vi "APC_PC_PythonGateway.vi"() -> ()   [LabVIEW 2020]
uses:
  controls/APC_ControlSettings.ctl
  controls/APC_PIDcontrolSettings.ctl
panel:
  out "System State 2":i8
  in  "stop":bool
  out "Client Connected":bool=TRUE
  out "Telemetry seq":i32
  out "Lines received":i32
  out "Last received":string
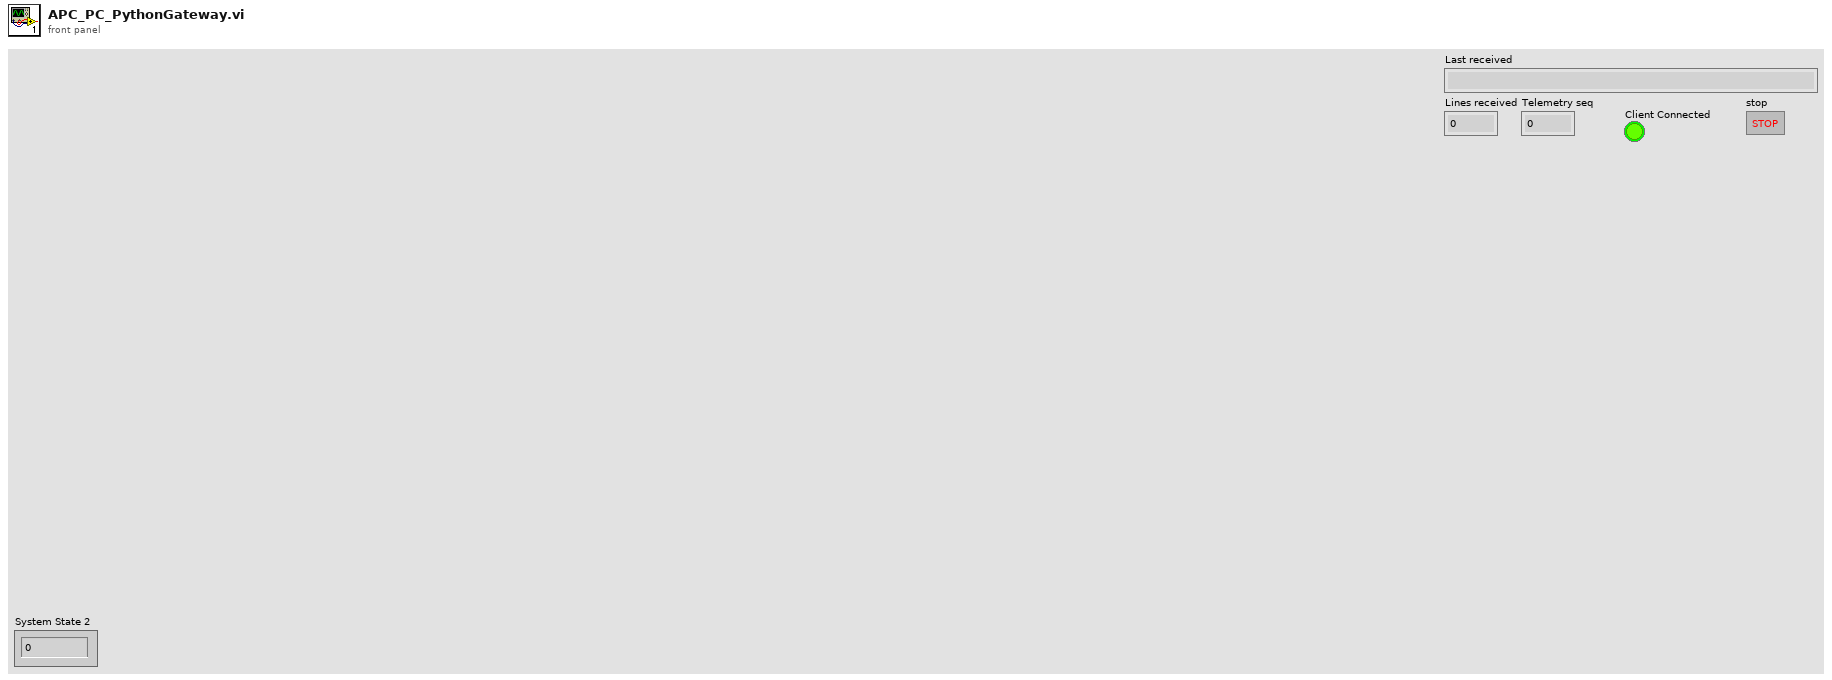
[diagram p1: front panel]
types:
  T1 = enum16{"Standard", "Buffered", "CRLF", "Immediate"}
  T2 = typedef "APC_ControlSettings.ctl" = cluster{"Spark advance [CADBTDC]":dbl, "Pref":dbl, "O2ref":dbl, "DI advance [CADBTDC]":dbl, "DI duration [ms] ":dbl, "CO2ref":dbl, "PFI duration [ms]":dbl, "IMEP ref":dbl, "Speed ref":dbl, "IGN enable":bool, "DI enable":bool, "CL PFI\n lambda":bool, "CL PFI\nIMEP":bool, "Activate\ncylinder":bool[], "Force idling":bool, "Force motoring":bool, "ETP resync":bool, "Requested mode":i8, "Clear Sync Errors":bool, "toggle TDC":bool, "l ref":dbl, "PID control references":T3, "CA50setpoint [CADATDC]":dbl, "CA50 control":bool, "Knock control":bool, "CLEAR EMERGENCY STOP":bool, "EMERGENCY STOP":bool}
  T3 = typedef "APC_PIDcontrolSettings.ctl" = cluster{"NG":bool, "Ar":bool, "O2":bool, "Intake vent":bool, "Cross vent":bool, "Exhaust vent":bool, "NG control mode":u8, "NG-FC-001-REF":dbl, "WF-OA-002-REF":dbl, "IMEP-REF":dbl, "Nm-REF":dbl, "Ar control mode":u8, "AR-PC-002-REF":dbl, "WF-PT-004-REF":dbl, "O2 control mode":u8, "O2-FC-001-REF":dbl, "WF-OA-001-REF":dbl, "Tcoolant control  mode":u8, "EC-FC-001-REF":dbl, "EC-TT-001-REF":dbl, "Texh control mode":u8, "SW-FC-004-REF":dbl, "SW-FT-002-REF":dbl, "WF-TT-004-REF":dbl, "Toil control mode":u8, "SW-FC-009-REF":dbl, "SW-FT-004-REF":dbl, "EO-TT-001-REF":dbl, "AIC201_CO2_ConcTarget":dbl, "O2_FF_NG":bool, "Dyno control mode":u8, "Membrane control mode":u8, "AR-FT-001-REF":dbl, "MTR modbus floats":sgl[], "MTR modbus u16":u16[], "MTR HB":bool, "PC_HB":bool, "EMERGENCY STOP":bool}
  T4 = cluster{"Spark advance [CADBTDC]":dbl, "Pref":dbl, "O2ref":dbl, "DI advance [CADBTDC]":dbl, "DI duration [ms] ":dbl, "CO2ref":dbl, "PFI duration [ms]":dbl, "IMEP ref":dbl, "Speed ref":dbl, "IGN enable":bool, "DI enable":bool, "CL PFI\n lambda":bool, "CL PFI\nIMEP":bool, "Activate\ncylinder":bool[], "Force idling":bool, "Force motoring":bool, "ETP resync":bool, "Requested mode":i8, "Clear Sync Errors":bool, "toggle TDC":bool, "l ref":dbl, "PID control references":T3, "CA50setpoint [CADATDC]":dbl, "CA50 control":bool, "Knock control":bool, "CLEAR EMERGENCY STOP":bool, "EMERGENCY STOP":bool}
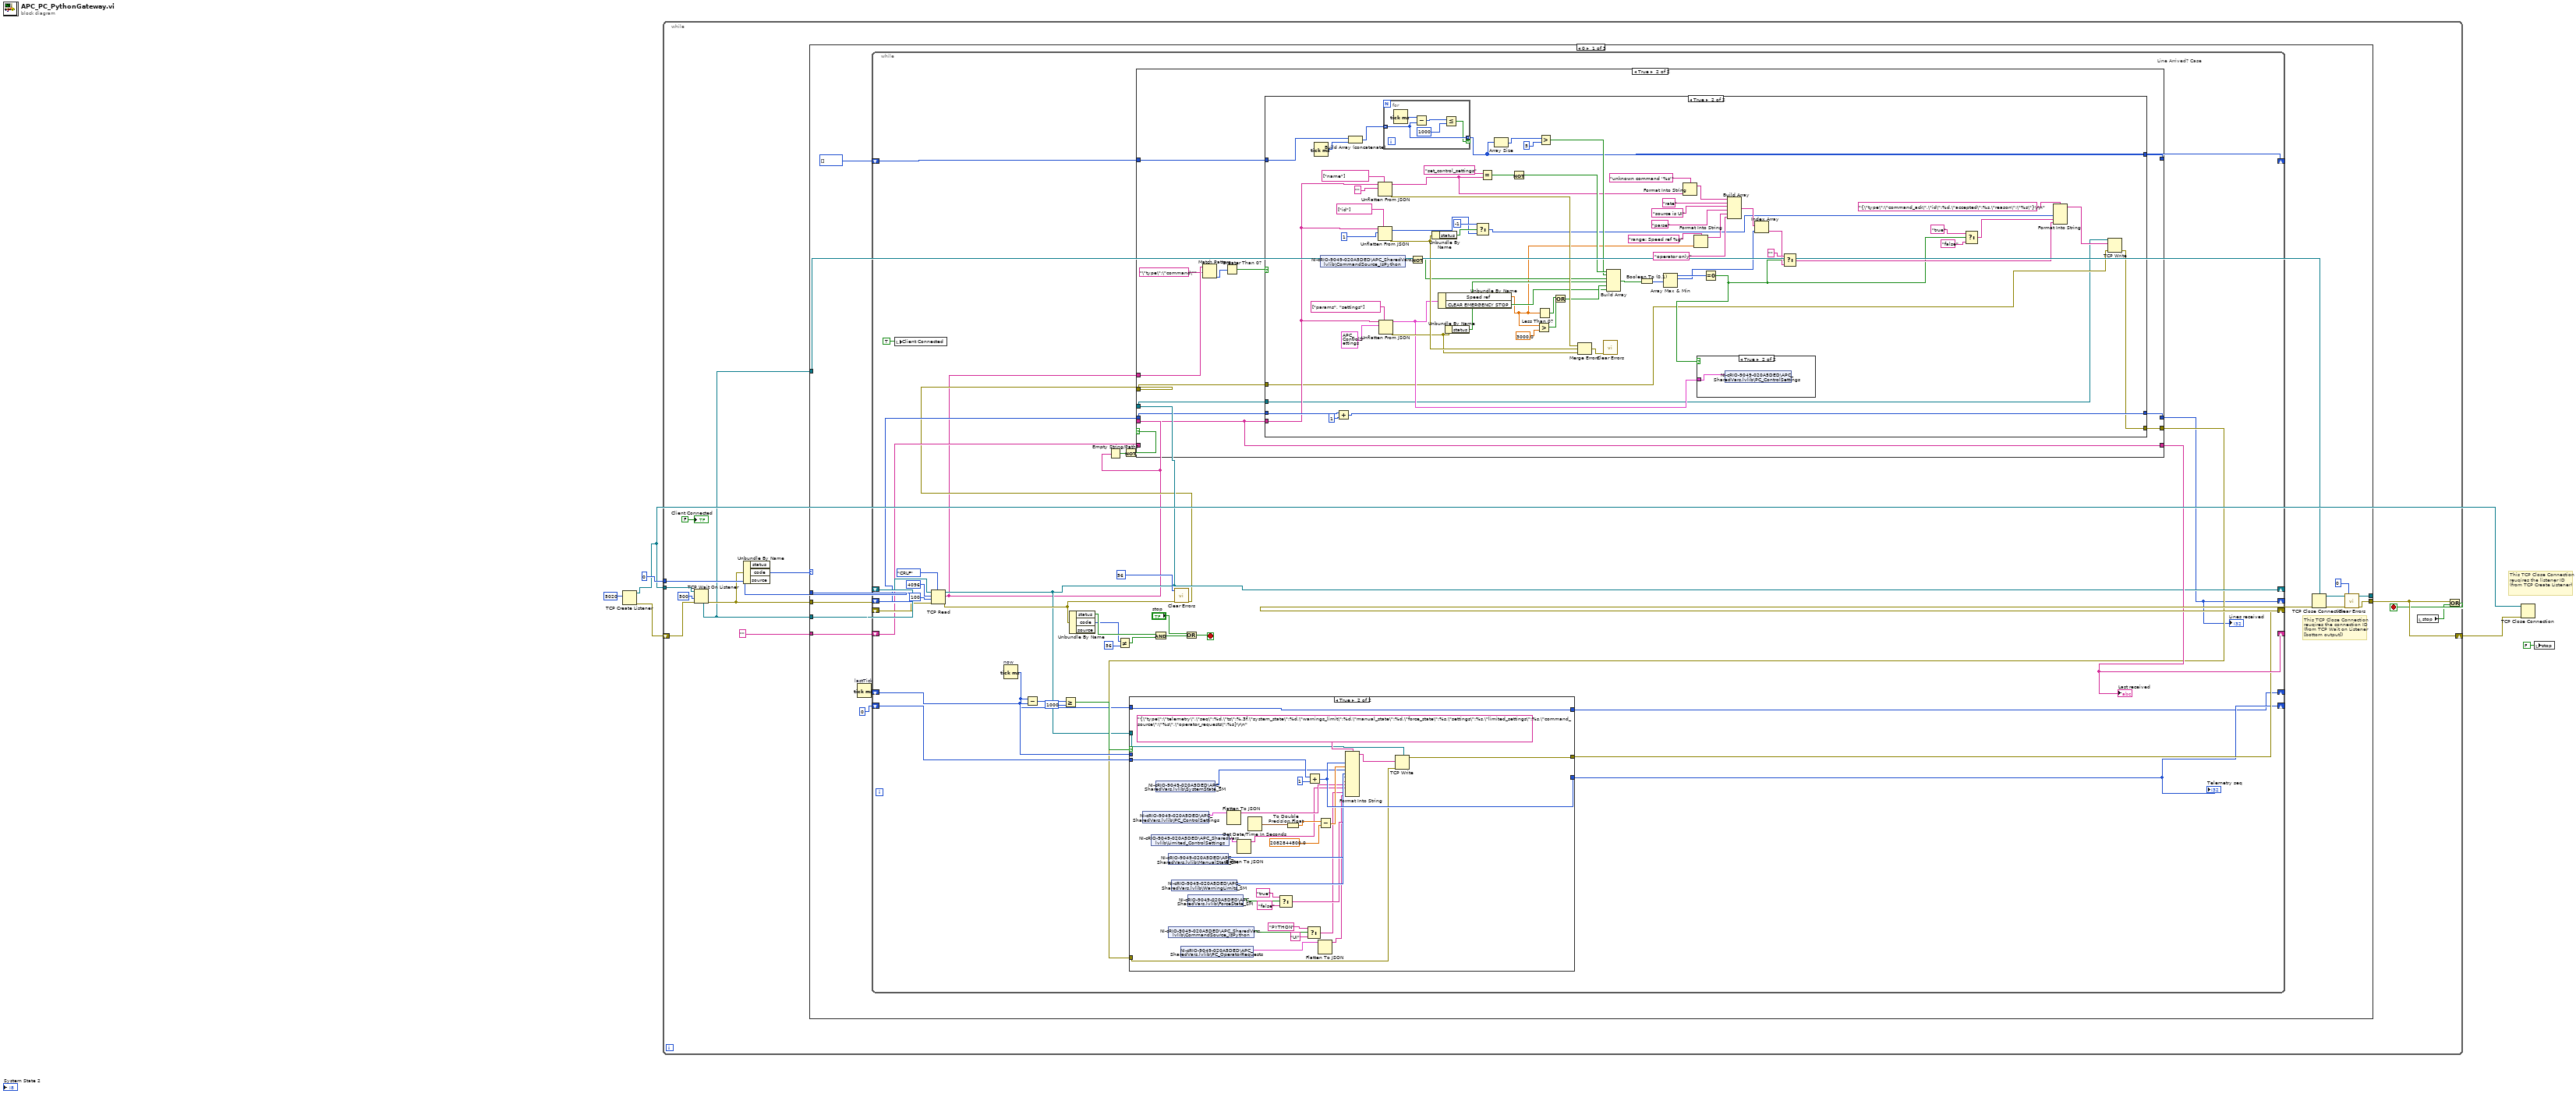
[diagram p0: block diagram]
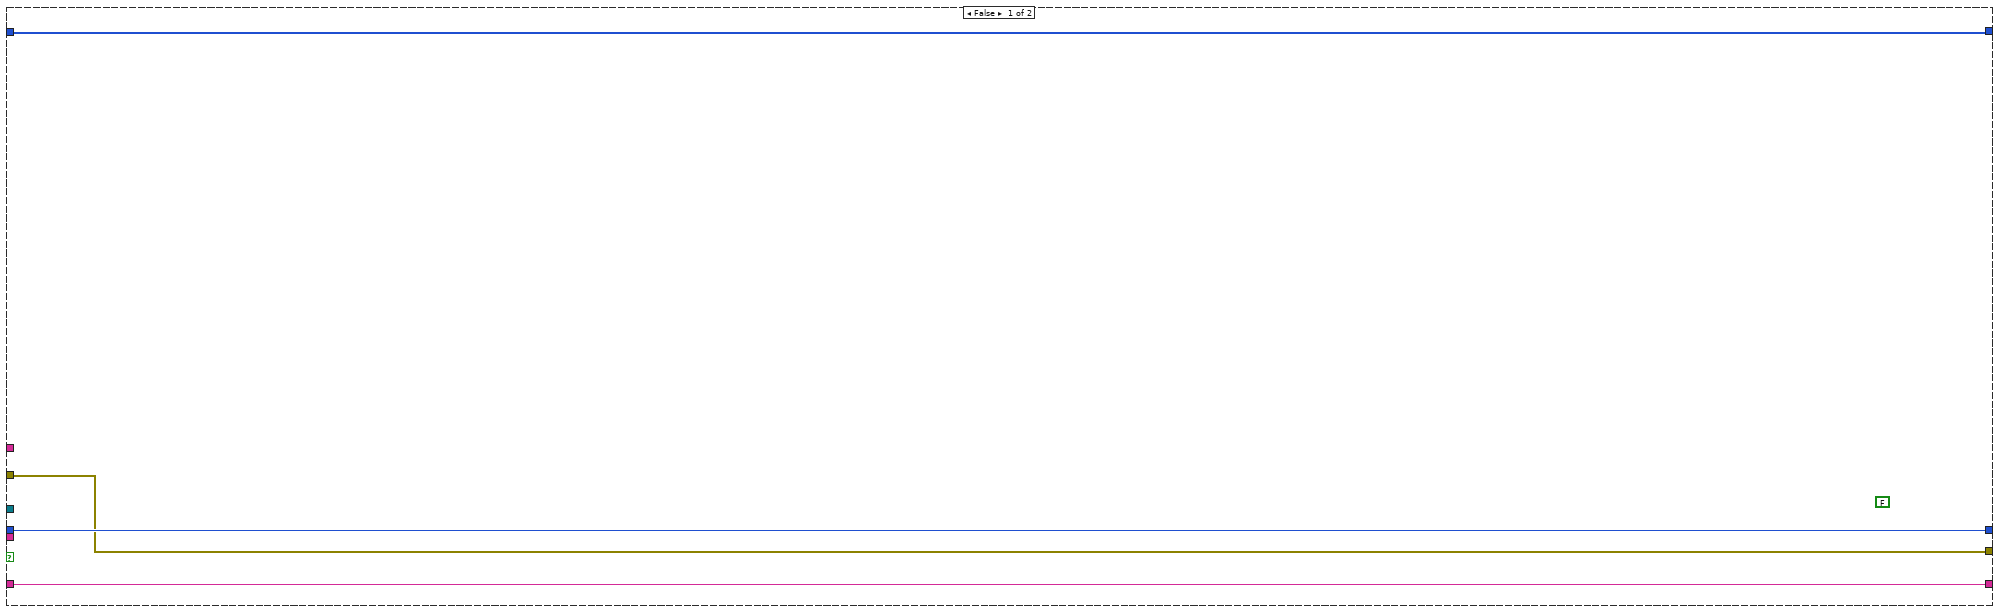
[diagram p3: hidden frame]
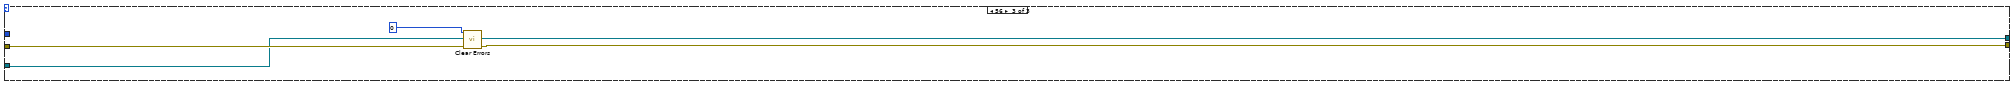
[diagram p7: hidden frame]
diagram:
  # "This TCP Close Connection reuqires the listener ID (from TCP Create Listener)"
  n1 = TCP Create Listener(10:u16 5020 ("port")) -> (0:w4:errorcluster, 3:w1:refnum<k5>)  [unwired: 4 in, 1 out]
  n2 = while {
    tunnel: 0 ("Lines received") -> [w17]
    shift-right: [w12] -> w3
    shift-left: w4 -> [w16]
    tunnel: w1 -> [w9]
    stop <- w11 stop-if-true
    n3 = TCP Wait On Listener(8:w16, 9:500 ("timeout ms (wait forever: -1)"), 11:w9) -> (0:w14:errorcluster, 4:w8:refnum<k5>)  [unwired: 1 in, 3 out]
    n4 = Unbundle By Name(w14) -> ("code"=w13:i32)  [unwired: 2 out]
    n5 = case shown="0" w13 {
      tunnel: w8 -> [w31 w191 w192]
      tunnel: w17 -> [w30 _ _]
      tunnel: [w24 w191 w192] -> _
      tunnel: [w25 w190 w193] -> w12
      tunnel: w14 -> [w29 w190 w194]
      tunnel: w8 -> [w23 _ _]
      tunnel: "" -> [w22 _ _]
      frame 0 {
        # "This TCP Close Connection reuqires the connection ID (from TCP Wait on Listener [bottom output])"
        n6 = Tick Count (ms) "lastTick"() -> (millisecond timer value=w21:u32)
        n7 = while {
          shift-right: [w33] -> _
          shift-left: w30 -> [w58]
          shift-right: [w53] -> w28
          shift-left: w29 -> [w61]
          shift-right: [w38] -> _
          shift-left: w31 -> [w67]
          shift-right: [w59] -> _
          shift-left: w22 -> [w60]
          shift-right: [w51] -> _
          shift-left: w21 -> [w50]
          shift-right: [w52] -> _
          shift-left: 0 -> [w54]
          shift-right: [w39] -> _
          shift-left: u32[] [] -> [w40]
          stop <- w47 stop-if-true
          n8 = local write "Client Connected"(TRUE ("Client Connected")) -> ()
          n9 = TCP Read(connection ID=w67, bytes to read=4096, error in (no error)=w61, 7:T1."CRLF" ("mode (standard)"), 9:100 ("timeout ms (25000)")) -> (connection ID out=w38:refnum<k5>, data out=w32:string, error out=w48:errorcluster)
          n10 = Tick Count (ms) "now"() -> (millisecond timer value=w49:u32)
          n11 = Subtract(x=w49, y=w50) -> (x-y=w57:u32)
          n12 = Greater Or Equal?(x=w57, y=u32 1000) -> (x >= y?=w55:bool)
          n13 = Unbundle By Name(w48) -> ("status"=w44:bool, "code"=w43:i32)  [unwired: 1 out]
          n14 = Empty String/Path?(string/path=w32) -> (empty?=w35:bool)
          n15 = Not Equal?(x=w43, y=56) -> (x != y?=w41:bool)
          n16 = Not(x=w35) -> (.not. x?=w34:bool)
          n17 = And(x=w44, y=w41) -> (x .and. y?=w45:bool)
          n18 = call <vilib>:"Clear Errors.vi"("error in (no error)"=w48, "specific error code to clear (0: all)"=56) -> ("error out"=w37:errorcluster)  [unwired: 4 in, 1 out]
          n19 = case "Line Arrived? Case" shown="True" w34 {
            tunnel: w60 -> [w104 _]
            tunnel: [w104 w112] -> w59
            tunnel: w32 -> [_ w112]
            tunnel: w58 -> [w103 w116]
            tunnel: [w103 w115] -> w33
            tunnel: [w102 w113] -> w39
            tunnel: w40 -> [w102 w114]
            tunnel: w38 -> [_ w109]
            tunnel: w37 -> [w101 w110]
            tunnel: [w101 w111] -> w36
            tunnel: w32 -> [_ w107]
            frame False {
              (unwired) FALSE
            }
            frame True {
              n20 = Match Pattern(string=w107, regular expression="\"type\":\"command\"") -> (offset past match=w108:i32)  [unwired: 1 in, 3 out]
              n21 = Greater Than 0?(x=w108) -> (x > 0?=w105:bool)
              n22 = case shown="True" w105 {
                tunnel: w116 -> [w118 w182]
                tunnel: [w118 w181] -> w115
                tunnel: w114 -> [w117 w157]
                tunnel: [w117 w154] -> w113
                tunnel: w112 -> [_ w134]
                tunnel: [w119 w125] -> w111
                tunnel: w110 -> [w119 w124]
                tunnel: w109 -> [_ w123]
                frame False {
                }
                frame True {
                  n23 = Tick Count (ms)() -> (millisecond timer value=w156:u32)
                  n24 = shared-variable "NI-cRIO-9049-020A5DED\\APC_SharedVars.lvlib\\CommandSource_IsPython"() -> (w153:bool)  [unwired: 1 in, 1 out]
                  n25 = Add(x=w182, y=1) -> (x+y=w181:i32)
                  n26 = Build Array (concatenate)(w157, w156) -> (w155:u32[])
                  n27 = Unflatten From JSON(path=string[] ["id"], JSON string=w134, type and defaults=1 ("y")) -> (value=w171:i32, error out=w169:errorcluster)  [unwired: 4 in]
                  n28 = Unflatten From JSON(path=string[] ["name"], JSON string=w134, type and defaults="") -> (value=w146:string, error out=w170:errorcluster)  [unwired: 4 in]
                  n29 = Unflatten From JSON(path=string[] ["params", "settings"], JSON string=w134, type and defaults=T2 {"Spark advance [CADBTDC]"=0.0, "Pref"=0.0, "O2ref"=0.0, "DI advance [CADBTDC]"=0.0, "DI duration [ms] "=0.0, "CO2ref"=0.0, "PFI duration [ms]"=0.0, "IMEP ref"=0.0, "Speed ref"=1800.0, "IGN enable"=TRUE, "DI enable"=TRUE, "CL PFI\n lambda"=FALSE, "CL PFI\nIMEP"=FALSE, "Activate\ncylinder"=[FALSE, FALSE, FALSE, FALSE, FALSE, FALSE], "Force idling"=FALSE, "Force motoring"=FALSE, "ETP resync"=FALSE, "Requested mode"=0, "Clear Sync Errors"=FALSE, "toggle TDC"=FALSE, "l ref"=0.0, "PID control references"={"NG"=FALSE, "Ar"=FALSE, "O2"=FALSE, "Intake vent"=FALSE, "Cross vent"=FALSE, "Exhaust vent"=FALSE, "NG control mode"=0, "NG-FC-001-REF"=0.0, "WF-OA-002-REF"=0.0, "IMEP-REF"=0.0, "Nm-REF"=0.0, "Ar control mode"=0, "AR-PC-002-REF"=0.0, "WF-PT-004-REF"=0.0, "O2 control mode"=0, "O2-FC-001-REF"=0.0, "WF-OA-001-REF"=0.0, "Tcoolant control  mode"=0, "EC-FC-001-REF"=0.0, "EC-TT-001-REF"=0.0, "Texh control mode"=0, "SW-FC-004-REF"=0.0, "SW-FT-002-REF"=0.0, "WF-TT-004-REF"=0.0, "Toil control mode"=0, "SW-FC-009-REF"=0.0, "SW-FT-004-REF"=0.0, "EO-TT-001-REF"=0.0, "AIC201_CO2_ConcTarget"=0.0, "O2_FF_NG"=FALSE, "Dyno control mode"=0, "Membrane control mode"=0, "AR-FT-001-REF"=0.0, "MTR modbus floats"=[0.0, 0.0, 0.0, 0.0, 0.0, 0.0, 0.0, 0.0, 0.0, 0.0, 0.0, 0.0, 0.0, 0.0, 0.0, 0.0, 0.0, 0.0, 0.0], "MTR modbus u16"=[0, 0, 0, 0, 0, 0, 0], "MTR HB"=FALSE, "PC_HB"=FALSE, "EMERGENCY STOP"=FALSE}, "CA50setpoint [CADATDC]"=0.0, "CA50 control"=TRUE, "Knock control"=FALSE, "CLEAR EMERGENCY STOP"=FALSE, "EMERGENCY STOP"=FALSE} ("APCControlSettings")) -> (value=w133:T2, error out=w168:errorcluster)  [unwired: 4 in]
                  n30 = for {
                    tunnel: w155 -> [w186] mode=indexing
                    tunnel: [w186] -> w154 mode=indexing if=w185
                    n31 = Tick Count (ms)() -> (millisecond timer value=w189:u32)
                    n32 = Subtract(x=w189, y=w186) -> (x-y=w188:u32)
                    n33 = Less Or Equal?(x=w188, y=u32 1000) -> (x <= y?=w185:bool)
                  }
                  n34 = Not(x=w153) -> (.not. x?=w152:bool)
                  n35 = Unbundle By Name(w169) -> ("status"=w173:bool)
                  n36 = Unbundle By Name(w133) -> ("Speed ref"=w145:dbl, "CLEAR EMERGENCY STOP"=w150:bool)
                  n37 = Unbundle By Name(w168) -> ("status"=w164:bool)
                  n38 = Select(t=-1, s=w173, f=w171) -> (s? t:f=w131:i32)
                  n39 = Equal?(x="set_control_settings", y=w146) -> (x = y?=w166:bool)
                  n40 = Array Size(array=w154) -> (size(s)=w162:i32)
                  n41 = Not(x=w166) -> (.not. x?=w165:bool)
                  n42 = Greater?(x=w145, y=3000.0) -> (0:w158:bool)
                  n43 = Less Than 0?(x=w145) -> (x < 0?=w160:bool)
                  n44 = Greater?(x=w162, y=5) -> (0:w161:bool)
                  n45 = Or(x=w160, y=w158) -> (x .or. y?=w159:bool)
                  n46 = Merge Errors(w170, w169, w168) -> (w167:errorcluster)
                  n47 = call <vilib>:"Clear Errors.vi"("error in (no error)"=w167) -> ()  [unwired: 5 in, 2 out]
                  n48 = Build Array(w165, w161, w152, w164, w159, w150) -> (w149:bool[])
                  n49 = Boolean To (0,1)(Boolean=w149) -> (0, 1=w148:i16[])
                  n50 = Array Max & Min(array=w148) -> (max value=w147:i16, max index (indices)=w137:i32)  [unwired: 2 out]
                  n51 = Format Into String(format string="unknown command '%s'" ("initial string"), w146) -> (resulting string=w144:string)  [unwired: 2 in, 1 out]
                  n52 = Format Into String(format string="range: Speed ref %g" ("initial string"), w145) -> (resulting string=w140:string)  [unwired: 2 in, 1 out]
                  n53 = Equal To 0?(x=w147) -> (x = 0?=w130:bool)
                  n54 = case shown="True" w130 {
                    tunnel: w133 -> [_ w184]
                    frame False {
                    }
                    frame True {
                      n55 = shared-variable "NI-cRIO-9049-020A5DED\\APC_SharedVars.lvlib\\PC_ControlSettings"(w184) -> ()  [unwired: 1 in, 1 out]
                    }
                  }
                  n56 = Build Array(w144, "rate", "source is UI", "parse", w140, "operator only") -> (w138:string[])
                  n57 = Index Array(array=w138, index=w137) -> (element=w135:string)
                  n58 = Select(t="", s=w130, f=w135) -> (s? t:f=w132:string)
                  n59 = Select(t="true", s=w130, f="false") -> (s? t:f=w127:string)
                  n60 = Format Into String(format string="{\"type\":\"command_ack\",\"id\":%d,\"accepted\":%s,\"reason\":\"%s\"}\r\n", w131, w127, w132) -> (resulting string=w126:string)  [unwired: 2 in, 1 out]
                  n61 = TCP Write(connection ID=w123, data in=w126, error in (no error)=w124) -> (error out=w125:errorcluster)  [unwired: 1 in, 2 out]
                }
              }
            }
          }
          "Last received" <- w59
          "Lines received" <- w33
          n62 = case shown="True" w55 {
            tunnel: w54 -> [w70 w88]
            tunnel: [w70 w98] -> w52
            tunnel: w38 -> [_ w96]
            tunnel: w36 -> [w69 w95]
            tunnel: [w69 w94] -> w53
            tunnel: [w68 w93] -> w51
            tunnel: w50 -> [w68 _]
            tunnel: w49 -> [_ w93]
            frame False {
            }
            frame True {
              n63 = shared-variable "NI-cRIO-9049-020A5DED\\APC_SharedVars.lvlib\\PC_ControlSettings"() -> (w87:T2)  [unwired: 1 in, 1 out]
              n64 = shared-variable "NI-cRIO-9049-020A5DED\\APC_SharedVars.lvlib\\Limited_ControlSettings"() -> (w86:T4)  [unwired: 1 in, 1 out]
              n65 = shared-variable "NI-cRIO-9049-020A5DED\\APC_SharedVars.lvlib\\SystemState_SM"() -> (w77:i8)  [unwired: 1 in, 1 out]
              n66 = shared-variable "NI-cRIO-9049-020A5DED\\APC_SharedVars.lvlib\\ManualState_SM"() -> (w84:i8)  [unwired: 1 in, 1 out]
              n67 = shared-variable "NI-cRIO-9049-020A5DED\\APC_SharedVars.lvlib\\CommandSource_IsPython"() -> (w76:bool)  [unwired: 1 in, 1 out]
              n68 = shared-variable "NI-cRIO-9049-020A5DED\\APC_SharedVars.lvlib\\WarningLimits_SM"() -> (w85:i8)  [unwired: 1 in, 1 out]
              n69 = shared-variable "NI-cRIO-9049-020A5DED\\APC_SharedVars.lvlib\\PC_OperatorRequests"() -> (w72:T2)  [unwired: 1 in, 1 out]
              n70 = shared-variable "NI-cRIO-9049-020A5DED\\APC_SharedVars.lvlib\\ForceState_SM"() -> (w81:bool)  [unwired: 1 in, 1 out]
              n71 = Flatten To JSON(anything=w87) -> (JSON string=w83:string)  [unwired: 2 in, 1 out]
              n72 = Flatten To JSON(anything=w86) -> (JSON string=w82:string)  [unwired: 2 in, 1 out]
              n73 = Get Date/Time In Seconds() -> (seconds since 1Jan1904=w92:timestamp)
              n74 = Select(t="true", s=w81, f="false") -> (s? t:f=w78:string)
              n75 = To Double Precision Float(number=w92) -> (double precision float=w91:dbl)
              n76 = Select(t="PYTHON", s=w76, f="UI") -> (s? t:f=w73:string)
              n77 = Add(x=w88, y=1) -> (x+y=w98:i32)
              n78 = Flatten To JSON(anything=w72) -> (JSON string=w71:string)  [unwired: 2 in, 1 out]
              n79 = Subtract(x=w91, y=2082844800.0) -> (x-y=w89:dbl)
              n80 = Format Into String(format string="{\"type\":\"telemetry\",\"seq\":%d,\"ts\":%.3f,\"system_state\":%d,\"warnings_limit\":%d,\"manual_state\":%d,\"force_state\":%s,\"settings\":%s,\"limited_settings\":%s,\"command_source\":\"%s\",\"operator_requests\":%s}\r\n", w98, w89, w77, w85, w84, w78, w83, w82, w73, w71) -> (resulting string=w97:string)  [unwired: 2 in, 1 out]
              n81 = TCP Write(connection ID=w96, data in=w97, error in (no error)=w95) -> (error out=w94:errorcluster)  [unwired: 1 in, 2 out]
            }
          }
          "Telemetry seq" <- w52
          n82 = Or(x="stop", y=w45) -> (x .or. y?=w47:bool)
        }
        n83 = TCP Close Connection(connection ID=w23, error in (no error)=w28) -> (connection ID out=w24:refnum<k5>, error out=w27:errorcluster)  [unwired: 1 in]
        n84 = call <vilib>:"Clear Errors.vi"("error in (no error)"=w27, "specific error code to clear (0: all)"=0) -> ("error out"=w25:errorcluster)  [unwired: 4 in, 1 out]
      }
      frame Default {
      }
      frame 56 {
        n85 = call <vilib>:"Clear Errors.vi"("error in (no error)"=w194, "specific error code to clear (0: all)"=0) -> ("error out"=w193:errorcluster)  [unwired: 4 in, 1 out]
      }
    }
    n86 = local read "stop"() -> (w10:bool)
    n87 = Or(x=w12, y=w10) -> (x .or. y?=w11:bool)
    "Client Connected" <- FALSE ("Client Connected")
  }
  n88 = TCP Close Connection(connection ID=w1, error in (no error)=w3) -> ()  [unwired: 1 in, 2 out]
  n89 = local write "stop"(FALSE ("stop")) -> ()
